vi "Create Frame (graphic).vi"(6 "stylename":string, 8 "error in (no error)":errorcluster, 9 "drawName":string, 10 "Graphic file":path, 11 "ooWriter in":refnum<class "ooWriter.lvclass">) -> (0 "error out":errorcluster, 2 "Frame (graphic)":refnum<k24>, 3 "ooWriter out":refnum<class "ooWriter.lvclass">)   [LabVIEW 2009, in "ooWriter.lvclass"]
uses:
  ooWriter.lvclass
  C:/Projets/LAVAG/OpenOfficeRGT/AODL/DLLs/AODL.dll
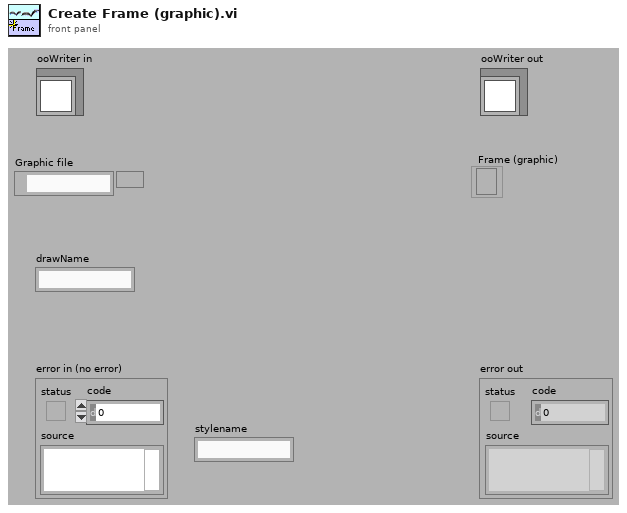
[diagram p1: front panel]
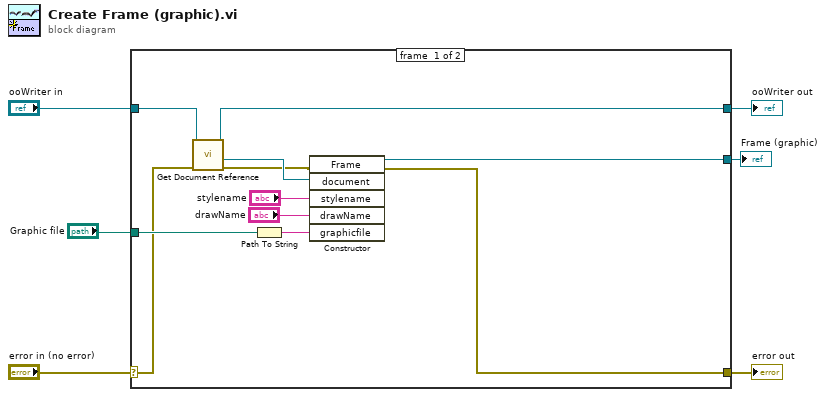
[diagram p0: block diagram]
diagram:
  n1 = case shown="No Error" "error in (no error)" {
    selector: "error in (no error)" -> [w8 w19]
    tunnel: [w7 w19] -> w5
    tunnel: [w10 w18] -> w3
    tunnel: "ooWriter in" -> [w11 w18]
    tunnel: "Graphic file" -> [w17 _]
    tunnel: [w13 _] -> w1
    frame #0 {
      n2 = call-dynamic "Get Document Reference.vi"("error in (no error)"=w8, "ooDocument in"=w11) -> ("error out"=w9:errorcluster, "Document"=w12:refnum<k24>, "ooDocument out"=w10:refnum<class "ooWriter.lvclass">)  [unwired: 7 in]
      n3 = Path To String(path=w17) -> (string=w16:string)
      n4 = constructor class="Frame"(error in=w9, "document"=w12, "stylename"="stylename", "drawName"="drawName", "graphicfile"=w16) -> (reference out=w13:refnum<k24>, error out=w7:errorcluster)  [unwired: 2 in, 5 out]
    }
    frame #1 {
    }
  }
  "error out" <- w5
  "ooWriter out" <- w3
  "Frame (graphic)" <- w1
